vi "3-state-control.vi"() -> ()   [LabVIEW 2024]
uses:
  ui-mode.ctl
  ui-mode-radio-button.ctl
panel:
  out "Numeric":dbl
  out "Test Mode Radio Button control 2":enum32{"Manual", "Cycle", "Auto Test"}(radio)
  in  "Test Mode Radio Button control":T1
  in  "C":bool
  in  "A":bool
  in  "B":bool
  in  "Stop Button":bool
  out "Bool State out":T2
  in  "Bool State in":T3
  # "Time On = 0 (always off)"
  # "Time On = 1 (always on)"
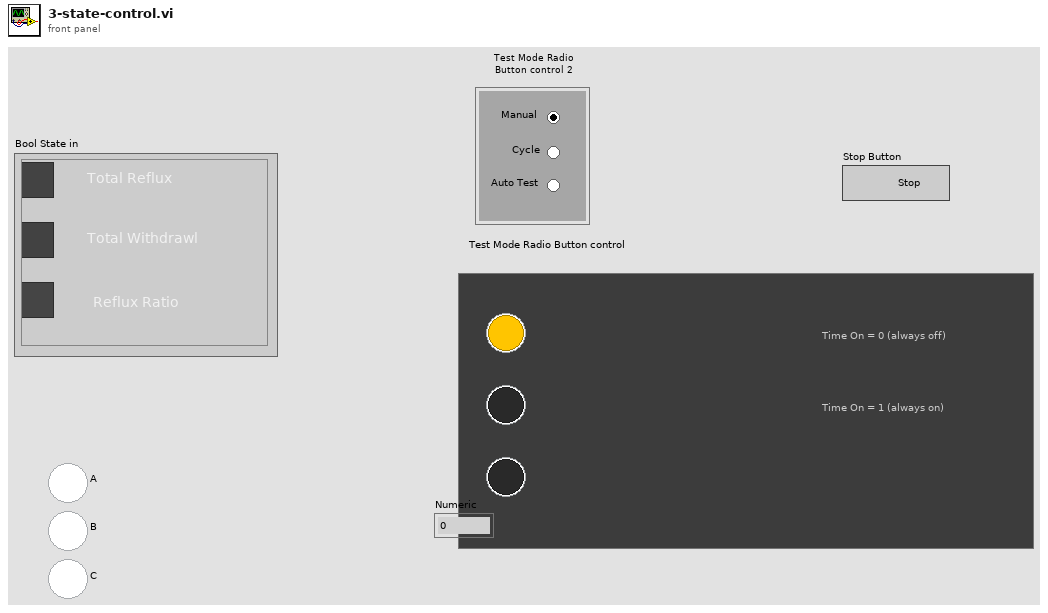
[diagram p1: front panel]
types:
  T1 = typedef "ui-mode-radio-button.ctl" = enum32{"    Total Reflux", "    Total Withdrawl", "    Reflux Ratio"}
  T2 = cluster{"Total Reflux":bool, "Total Withdrawl":bool, "Reflux Ratio":bool}
  T3 = typedef "ui-mode.ctl" = cluster{"Total Reflux":bool, "Total Withdrawl":bool, "Reflux Ratio":bool}
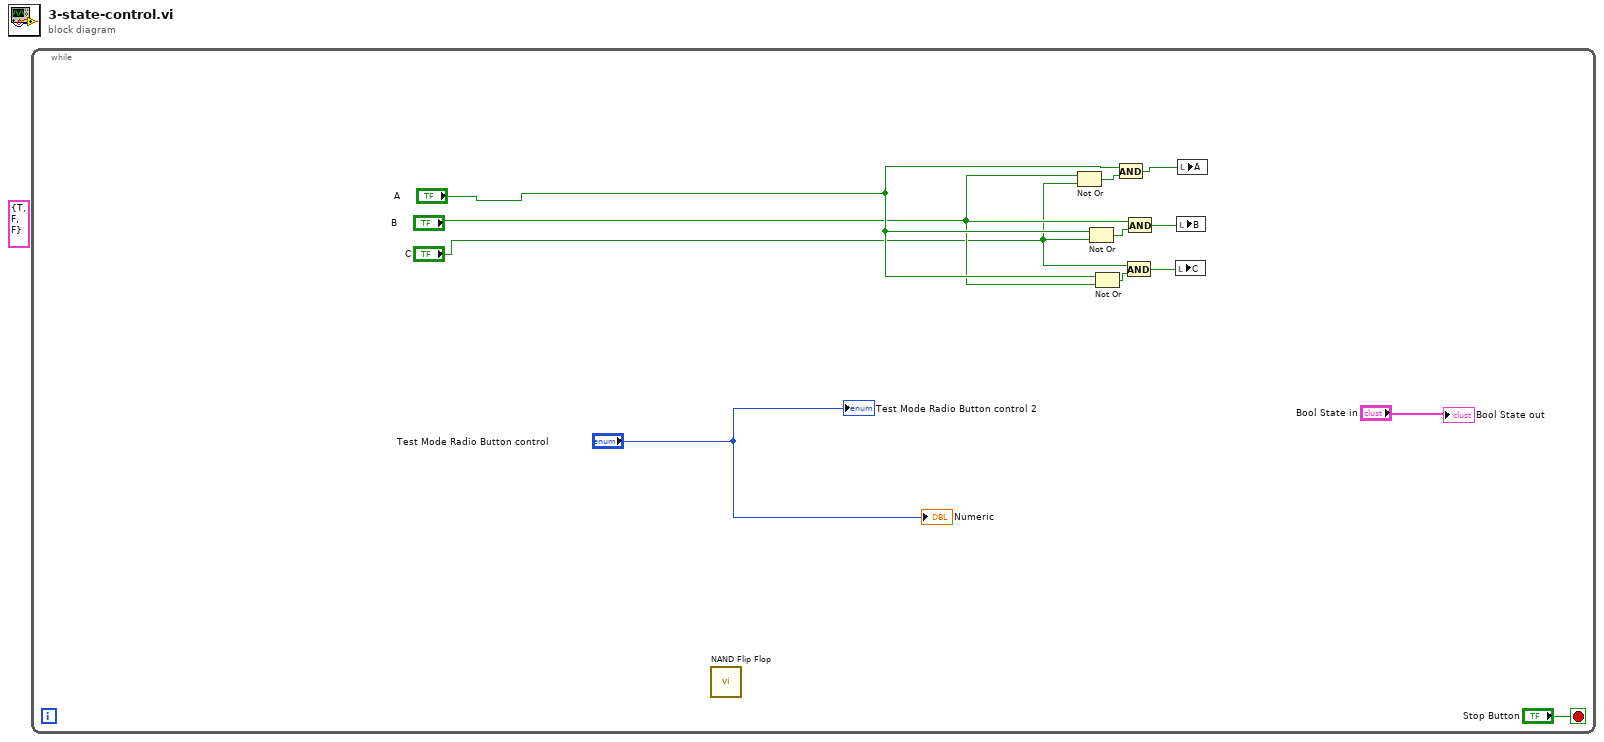
[diagram p0: block diagram]
diagram:
  (unwired) T2 {"Total Reflux"=TRUE, "Total Withdrawl"=FALSE, "Reflux Ratio"=FALSE} ("Bool State in")
  n1 = while {
    stop <- "Stop Button" stop-if-true
    n2 = call "NAND Flip Flop.vi"() -> ()  [unwired: 10 in, 2 out]
    n3 = Not Or(1:"C", 2:"B") -> (0:w11:bool)
    n4 = Not Or(1:"C", 2:"A") -> (0:w10:bool)
    n5 = Not Or(1:"B", 2:"A") -> (0:w9:bool)
    n6 = And(x="A", y=w11) -> (x .and. y?=w4:bool)
    n7 = And(x="C", y=w9) -> (x .and. y?=w2:bool)
    n8 = And(x="B", y=w10) -> (x .and. y?=w3:bool)
    n9 = local write "C"(w2) -> ()
    n10 = local write "B"(w3) -> ()
    n11 = local write "A"(w4) -> ()
    "Bool State out" <- "Bool State in"
    "Test Mode Radio Button control 2" <- "Test Mode Radio Button control"
    "Numeric" <- "Test Mode Radio Button control"
  }
